vi "Core Action.vi"(8 "error in (no error)":errorcluster, 10 "SECS-II Class":refnum<class "SECS-II Class.lvclass">, 11 "Host Requests Equipment Current Constant Values in":refnum<class "04-Host Requests Equipment Current Constant Values.lvclass">) -> (0 "error out":errorcluster, 2 "SECS-II Class Out":refnum<class "SECS-II Class.lvclass">, 3 "Host Requests Equipment Current Constant Values out":refnum<class "04-Host Requests Equipment Current Constant Values.lvclass">)   [LabVIEW 2020, in "SECS Scenarios.lvlib" / "04-Host Requests Equipment Current Constant Values.lvclass"]
uses:
  04-Host Requests Equipment Current Constant Values.lvclass
  D:/Dropbox/SECS/SECS_GEM v1.1.0/Com/SECS Scenarios/Scenarios Class/Scenarios Class.lvclass
  SECS Communication/SECS-II Class/SECS-II Class.lvclass
  SECS Communication/S2 Message Class/S2 Message Class.lvclass
  D:/Dropbox/SECS/SECS_GEM v1.1.0/Com/SECS Communication/SECS-II Class/SECS-II Class.lvclass
  Scenarios Class/Scenarios Class.lvclass/Scenarios Class.ctl
  Scenarios Class/Reply State.ctl
  SECS Communication/SECS-II Class/Format Code.ctl
  Scenarios Class/Write Reply State.vi
  Scenarios Class/Read HSMS Class.vi
  SECS Communication/SECS Data Class/Get ECID Data.vi
  SECS Communication/SECS Data Class/Get All ECID Data.vi
  SECS Communication/HSMS Class/HSMS Class.lvclass
  SECS Communication/SECS Data Class/SECS Data Class.lvclass
  Scenarios Class/Scenarios Class.lvclass
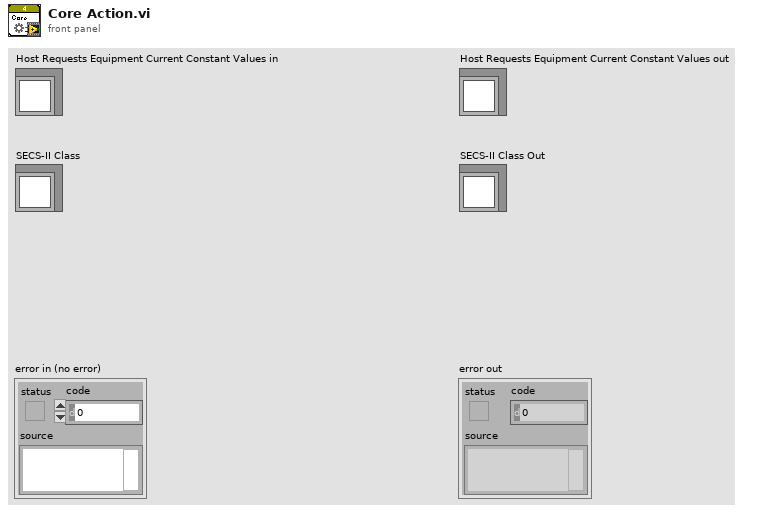
[diagram p1: front panel]
types:
  T1 = typedef "SECS Scenarios.lvlib/Scenarios Class.lvclass/Reply State.ctl" = enum16{"OK", "Illegal Data", "Unknown Stream", "Unknown Function", "Off-Line", "T3 Timeout", "Inner-Timeout"}
  T2 = typedef "SECS Communication.lvlib/SECS-II Class.lvclass/Format Code.ctl" = enum16{"L", "A", "B", "Boolean", "J", "I1", "I2", "I4", "I8", "U1", "U2", "U4", "U8", "F4", "F8", "Char"}
  T3 = typedef "SECS Communication.lvlib/SECS Data Class.lvclass/ECID Data.ctl" = cluster{"ECID":u32, "Name":string, "Description":string, "Format Code":T2, "Unit":string, "Max":dbl, "Min":dbl, "Default":string, "Source":string, "Data":variant}
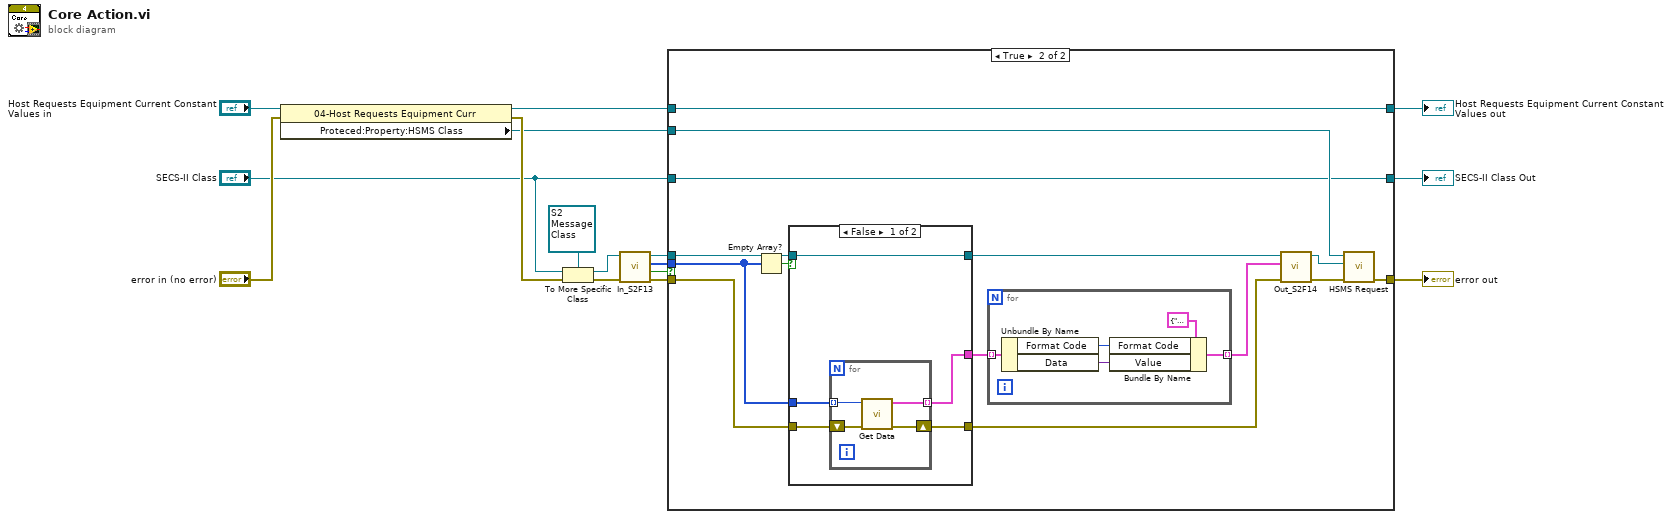
[diagram p0: block diagram]
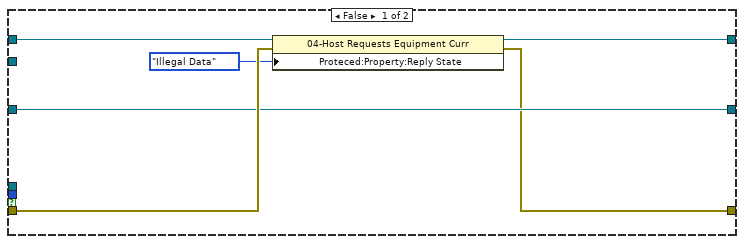
[diagram p2: hidden frame]
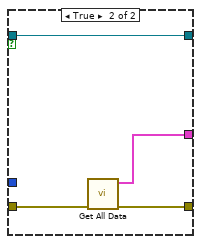
[diagram p3: hidden frame]
diagram:
  n1 = property class="04-Host Requests Equipment Curr"(reference="Host Requests Equipment Current Constant Values in", error in="error in (no error)") -> (reference out=w4:refnum<class "04-Host Requests Equipment Current Constant Values.lvclass">, error out=w16:errorcluster, "Proteced:Property:HSMS Class"=w15:refnum<class "HSMS Class.lvclass">)
  n2 = To More Specific Class(target class=refnum<class "S2 Message Class.lvclass"> refnum ("SECS Communication.lvlib:S2 Message Class.lvclass"), reference="SECS-II Class", error in=w16) -> (specific class reference=w11:refnum<class "S2 Message Class.lvclass">, error out=w12:errorcluster)
  n3 = call "In_S2F13.vi"("error in (no error)"=w12, "S2 Message Class in"=w11) -> ("error out"=w6:errorcluster, "OK?"=w5:bool, "Equipment Constant ID(ECID)"=w7:u32[], "S2 Message Class out"=w8:refnum<class "S2 Message Class.lvclass">)  [unwired: 6 in]
  n4 = case shown="True" w5 {
    tunnel: w15 -> [_ w36]
    tunnel: [w17 w33] -> w10
    tunnel: w8 -> [_ w30]
    tunnel: w7 -> [_ w29]
    tunnel: w6 -> [w21 w28]
    tunnel: w4 -> [w22 w24]
    tunnel: [w19 w24] -> w3
    tunnel: "SECS-II Class" -> [w18 w23]
    tunnel: [w18 w23] -> w1
    frame False {
      n5 = property class="04-Host Requests Equipment Curr"(reference=w22, error in=w21, "Proteced:Property:Reply State"=Reply_State."Illegal Data" ("Reply State")) -> (reference out=w19:refnum<class "04-Host Requests Equipment Current Constant Values.lvclass">, error out=w17:errorcluster)
    }
    frame True {
      n6 = Empty Array?(array=w29) -> (empty?=w31:bool)
      n7 = case shown="False" w31 {
        tunnel: w28 -> [w41 w49]
        tunnel: [w40 w47] -> w32
        tunnel: [w39 w48] -> w26
        tunnel: w29 -> [w38 _]
        tunnel: w30 -> [w37 w46]
        tunnel: [w37 w46] -> w27
        frame False {
          n8 = for {
            tunnel: w38 -> [w44] mode=indexing
            shift-right: [w43] -> w39
            shift-left: w41 -> [w45]
            tunnel: [w42] -> w40 mode=indexing
            n9 = call-poly "Get Data.vi"("error in"=w45, "ECID"=w44) -> ("error out"=w43:errorcluster, "ECID Data"=w42:T3)  [unwired: 7 in, 1 out]
          }
        }
        frame True {
          n10 = call-poly "Get All Data.vi"("error in (no error)"=w49) -> ("error out"=w48:errorcluster, "ECID Data"=w47:T3[])  [unwired: 9 in]
        }
      }
      n11 = for {
        tunnel: w32 -> [w54] mode=indexing
        tunnel: [w50] -> w25 mode=indexing
        n12 = Unbundle By Name(w54) -> ("Format Code"=w52:T2, "Data"=w51:variant)
        n13 = Bundle By Name(cluster=cluster{"Format Code":T2, "Value":variant} {"Format Code"=enum."A", "Value"=variant} ("SV"), "Format Code"=w52, "Value"=w51) -> (w50:cluster{"Format Code":T2, "Value":variant})
      }
      n14 = call "Out_S2F14.vi"("error in (no error)"=w26, "ECV"=w25, "S2 Message Class in"=w27) -> ("error out"=w34:errorcluster, "S2 Message Class out"=w35:refnum<class "S2 Message Class.lvclass">)  [unwired: 7 in]
      n15 = call "HSMS Request.vi"("error in (no error)"=w34, "SECS-II Class In"=w35, "HSMS Class in"=w36) -> ("error out"=w33:errorcluster)  [unwired: 7 in, 1 out]
    }
  }
  "error out" <- w10
  "Host Requests Equipment Current Constant Values out" <- w3
  "SECS-II Class Out" <- w1
